vi "Init Hardware.vi"(8 "error in (no error)":errorcluster, 11 "RFSoC Driver in":refnum<class "RFSoC Driver.lvclass">) -> (0 "error out":errorcluster, 3 "RFSoC Driver out":refnum<class "RFSoC Driver.lvclass">)   [LabVIEW 2020, in "RFSoC Driver.lvclass"]
uses:
  RFSoC Driver.lvclass
  RFSoC Driver.lvclass/RFSoC Driver.ctl
  Read address.vi
  Pulse Driver/Pulse Driver.lvclass
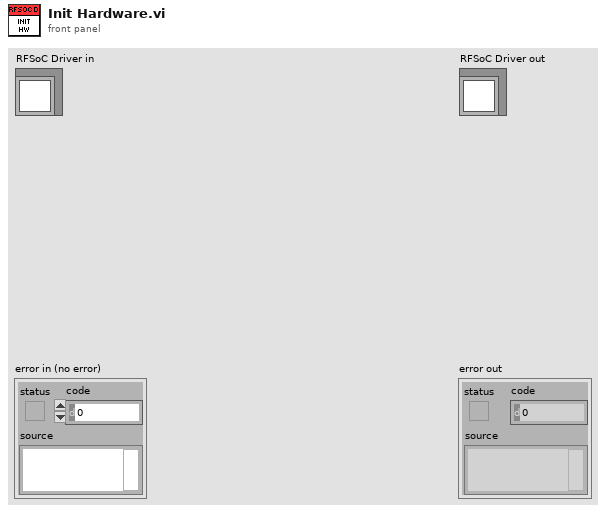
[diagram p1: front panel]
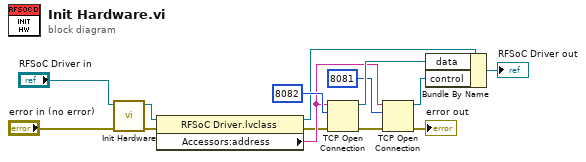
[diagram p0: block diagram]
diagram:
  n1 = call-parent "Init Hardware.vi"("error in (no error)"="error in (no error)", "Instrument Driver in"="RFSoC Driver in") -> ("error out"=w14:errorcluster, "Instrument Driver out"=w10:refnum<class "RFSoC Driver.lvclass">)  [unwired: 8 in]
  n2 = property class="RFSoC Driver.lvclass"(reference=w10, error in=w14) -> (reference out=w9:refnum<class "RFSoC Driver.lvclass">, error out=w3:errorcluster, "Accessors:address"=w4:string)
  n3 = TCP Open Connection(address=w4, remote port or service name=u16 8082, error in (no error)=w3) -> (connection ID=w7:refnum<k5>, error out=w5:errorcluster)  [unwired: 2 in]
  n4 = TCP Open Connection(address=w4, remote port or service name=u16 8081, error in (no error)=w5) -> (connection ID=w1:refnum<k5>, error out=→"error out":errorcluster)  [unwired: 2 in]
  n5 = Bundle By Name(cluster=w9, "data"=w7, "control"=w1) -> (→"RFSoC Driver out":refnum<class "RFSoC Driver.lvclass">)
